vi "Joystick.vi"(10 "Refnum Name":string, 11 "JoystickDevice":T1) -> (0 "error out":errorcluster, 1 "Buttons":bool[](array[boolean]), 2 "Axes":dbl[](array[numeric]))   [LabVIEW 2018]
uses:
  <vilib>/Rock Robotics/WPI/Joystick/WPI_JoystickDeviceEnum.ctl
  <vilib>/Rock Robotics/Network Tables/NT Write Numeric Array.vi
  <vilib>/Rock Robotics/Network Tables/NT Write Boolean Array.vi
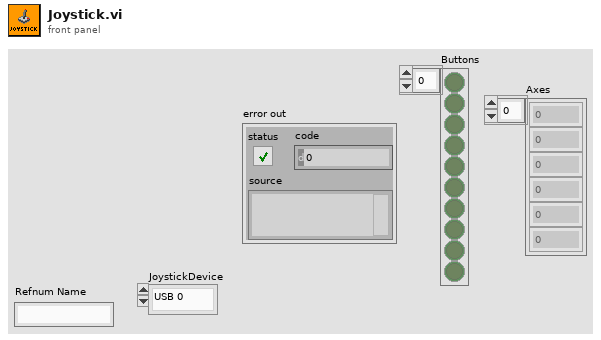
[diagram p1: front panel]
types:
  T1 = typedef "WPI_JoystickDeviceEnum.ctl" = enum16{"USB 0", "USB 1", "USB 2", "USB 3", "USB 4", "USB 5"}
  T2 = typedef "WPI_Joystick Info.ctl" = cluster{"Device Name":string, "HID Type":T3, "XBox Type":T4, "Axes Count":i32, "Axes Types":T5[], "Button Count":i32, "POV Count":i32}
  T3 = typedef "WPI_JoystickHID Types.ctl" = enum16{"Not HID", "HID Joystick", "HID Gamepad", "HID Driving Wheel", "HID Flightstick", "HID First Person"}
  T4 = typedef "WPI_JoystickXBox Types.ctl" = enum16{"Not XBox", "XBox Unknown", "XBox Gamepad", "XBox Wheel", "XBox Arcade Stick", "XBox Flight Stick", "XBox Dance Pad", "XBox Guitar", "XBox Drum Kit", "XBox Arcade Pad"}
  T5 = typedef "WPI_JoystickAxis Types.ctl" = enum16{"X Axis", "Y Axis", "Z Axis", "RxAxis", "RyAxis", "RzAxis", "Slider", "POV", "None", "L X Axis", "L Y Axis", "L Trigger", "R Trigger", "R X Axis", "R Y Axis"}
  T6 = typedef "WPI_JoystickDevRef.ctl" = cluster{"Device":T1}
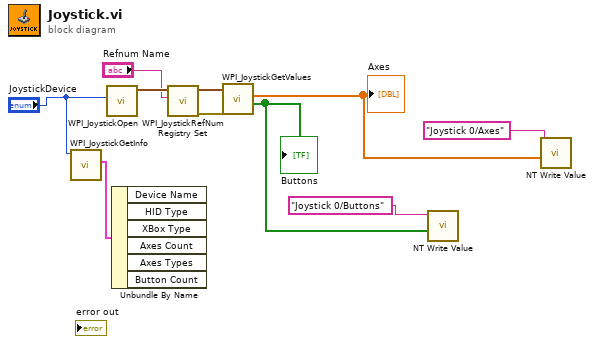
[diagram p0: block diagram]
diagram:
  n1 = call <vilib>:"WPI_JoystickGetInfo.vi"("JoystickDevice"="JoystickDevice") -> ("Joystick Info"=w10:T2)  [unwired: 9 in, 1 out]
  n2 = call <vilib>:"WPI_JoystickOpen.vi"("JoystickDevice"="JoystickDevice") -> ("JoystickDevRef"=w9:T6)  [unwired: 10 in]
  n3 = Unbundle By Name(w10) -> ()  [unwired: 6 out]
  n4 = call <vilib>:"WPI_JoystickRefNum Registry Set.vi"("refnum name"="Refnum Name", "JoystickDevRef"=w9) -> ("error out"=w6:errorcluster, "JoystickDevRef"=w5:T6)  [unwired: 8 in]
  n5 = call <vilib>:"WPI_JoystickGetValues.vi"("error in (no error)"=w6, "JoystickDevRef"=w5) -> ("Buttons"=w1:bool[], "Axes"=w3:dbl[])  [unwired: 5 in, 3 out]
  "Buttons" <- w1
  "Axes" <- w3
  n6 = call-poly <vilib>:"NT Write Value.vi"("Boolean Array"=w1, "Name"="Joystick 0/Buttons") -> ()  [unwired: 9 in, 1 out]
  n7 = call-poly <vilib>:"NT Write Value.vi"("Numeric Array"=w3, "Name"="Joystick 0/Axes") -> ()  [unwired: 9 in, 1 out]
